vi "Poll DMA.vi"(4 "Timeout is Error?":bool, 6 "Wait (ms)":u32=1, 8 "error in (no error)":errorcluster, 9 "Timeout (ms)":u32, 10 "Total Samples to Read":u32, 11 "DMA Ref":T1) -> (0 "error out":errorcluster, 3 "DMA Ref":T1, 5 "Timeout?":bool)   [LabVIEW 2016, in "FPGA Addon Engine.lvlib"]
uses:
  FPGA Addon Engine.lvlib
  Types/DMA Input Ref.ctl
  <vilib>/rvi/errors/niLvFpgaAdjustHostInterfaceError.vi
  <vilib>/Utility/error.llb/Error Cluster From Error Code.vi
  <vilib>/rvi/interface/nirviMethod/nirviMethod.xnode
  <vilib>/FPGAPlugInAG/Dynamic/niLvFpga_ReadFifo_Dynamic.vi
  <vilib>/rvi/errors/niLvFpgaMergeErrorWithErrorCode.vi
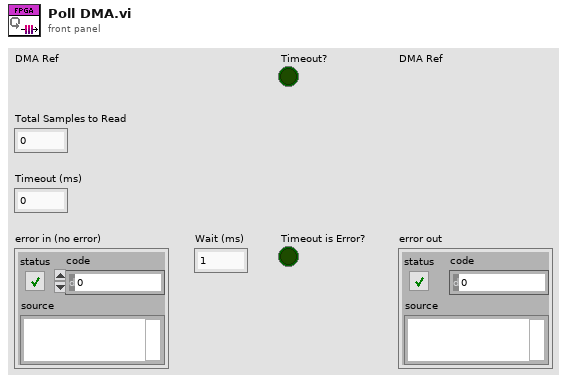
[diagram p1: front panel]
types:
  T1 = typedef "FPGA Addon Engine.lvlib/DMA Input Ref.ctl" = refnum<k20>
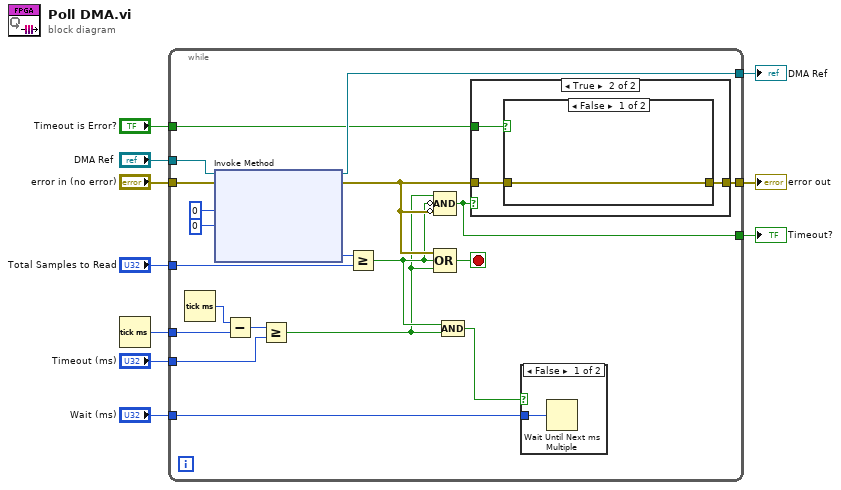
[diagram p0: block diagram]
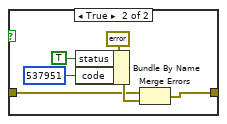
[diagram p4: hidden frame]
diagram:
  n1 = Tick Count (ms)() -> (millisecond timer value=w10:u32)
  n2 = while {
    tunnel: "error in (no error)" -> [w28]
    tunnel: "DMA Ref" -> [w27]
    tunnel: w10 -> [w25]
    tunnel: "Timeout (ms)" -> [w24]
    tunnel: [w23] -> w7
    tunnel: [w22] -> w8
    tunnel: "Total Samples to Read" -> [w20]
    tunnel: "Wait (ms)" -> [w19]
    tunnel: [w17] -> w2
    tunnel: "Timeout is Error?" -> [w16]
    stop <- w14 stop-if-true
    n3 = Tick Count (ms)() -> (millisecond timer value=w26:u32)
    n4 = xnode "Invoke Method"("FPGA VI Reference In"=w27, "error in"=w28, "Number of Elements"=u32 0, "Timeout (ms)"=0) -> ("FPGA VI Reference Out"=w22:T1, "error out"=w15:errorcluster, "Elements Remaining"=w21:u32)  [unwired: 1 out]
    n5 = Subtract(x=w26, y=w25) -> (x-y=w18:u32)
    n6 = Greater Or Equal?(x=w18, y=w24) -> (x >= y?=w12:bool)
    n7 = Greater Or Equal?(x=w21, y=w20) -> (x >= y?=w13:bool)
    n8 = Compound Arithmetic op=AND(w12, invert w13, invert w15) -> (w17:bool)
    n9 = Compound Arithmetic op=OR(w15, w13, w12) -> (w14:bool)
    n10 = Compound Arithmetic op=AND(w13, w12) -> (w11:bool)
    n11 = case shown="True" w17 {
      tunnel: w15 -> [w32 w35]
      tunnel: [w32 w34] -> w23
      tunnel: w16 -> [_ w33]
      frame False {
      }
      frame True {
        n12 = case shown="False" w33 {
          tunnel: w35 -> [w36 w39]
          tunnel: [w36 w38] -> w34
          frame False {
          }
          frame True {
            n13 = Bundle By Name(cluster=errorcluster {"status"=FALSE, "code"=0, "source"=""} ("error constant"), "status"=TRUE, "code"=537951) -> (w41:errorcluster)
            n14 = Merge Errors(w39, w41) -> (w38:errorcluster)
          }
        }
      }
    }
    n15 = case shown="False" w11 {
      tunnel: w19 -> [w31 _]
      frame False {
        n16 = Wait Until Next ms Multiple(millisecond multiple=w31) -> ()  [unwired: 1 out]
      }
      frame True {
      }
    }
  }
  "DMA Ref" <- w8
  "error out" <- w7
  "Timeout?" <- w2
